vi "FTW-Reply-Worker.vi"(1 "Endpoint":refnum<class "FTW-Endpoint.lvclass">, 2 "Message Handler":refnum<user-event>) -> ()   [LabVIEW 2013, in "FTW-Reply.lvclass"]
uses:
  FTW-Reply.lvclass
  Package/Request/FTW-Package-IncomingRequest.lvclass
  Endpoint/FTW-Endpoint.lvclass
panel:
  out "Messages Handled":u32
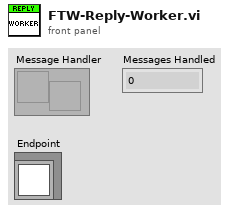
[diagram p1: front panel]
types:
  T1 = typedef "FTW-Message.ctl" = cluster{"Header":string, "Body":string, "Metadata":string}
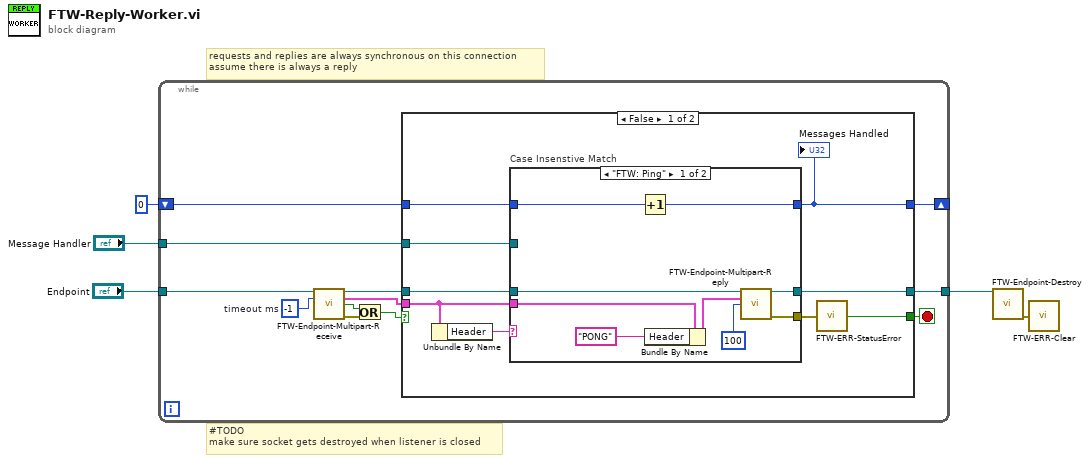
[diagram p0: block diagram]
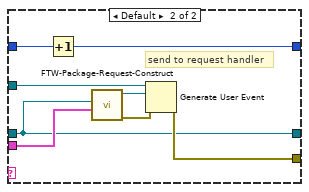
[diagram p2: hidden frame]
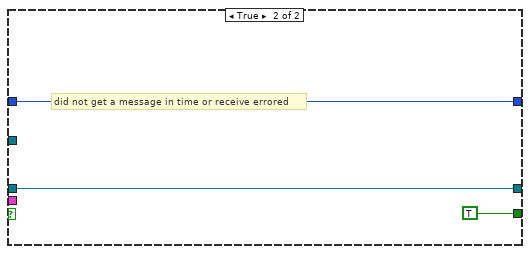
[diagram p3: hidden frame]
diagram:
  # "#TODO\nmake sure socket gets destroyed when listener is closed"
  # "requests and replies are always synchronous on this connection\nassume there is always a reply"
  n1 = while {
    tunnel: "Message Handler" -> [w17]
    shift-right: [w10] -> _
    shift-left: u32 0 -> [w11]
    tunnel: "Endpoint" -> [w16]
    tunnel: [w6] -> w3
    stop <- w12 stop-if-true
    w15 = -1  # timeout ms
    n2 = call-dynamic "FTW-Endpoint-Multipart-Receive.vi"("FTW Endpoint"=w16, "Timeout"=w15) -> ("FTW Endpoint out"=w9:refnum<class "FTW-Endpoint.lvclass">, "Message Received"=w13:T1, "Timed out?"=w7:bool, "error out"=w14:errorcluster)  [unwired: 10 in]
    n3 = Or(x=w7, y=w14) -> (x .or. y?=w8:bool)
    n4 = case shown="False" w8 {
      tunnel: w17 -> [w26 _]
      tunnel: w13 -> [w19 _]
      tunnel: [w22 TRUE] -> w12
      tunnel: w9 -> [w23 w44]
      tunnel: w11 -> [w25 w46]
      tunnel: [w20 w46] -> w10
      tunnel: [w21 w44] -> w6
      frame False {
        n5 = Unbundle By Name(w19) -> ("Header"=w18:string)
        n6 = case "Case Insenstive Match" shown="\"FTW: Ping\"" w18 {
          tunnel: w26 -> [_ w43]
          tunnel: w25 -> [w35 w42]
          tunnel: [w30 w41] -> w20
          tunnel: [w34 w38] -> w24
          tunnel: w23 -> [w33 w36]
          tunnel: w19 -> [w29 w37]
          tunnel: [w32 w36] -> w21
          frame "FTW: Ping" {
            n7 = Increment(x=w35) -> (x+1=w30:u32)
            n8 = Bundle By Name(cluster=w29, "Header"="PONG" ("Part")) -> (w28:T1)
            n9 = call-dynamic "FTW-Endpoint-Multipart-Reply.vi"("FTW Endpoint"=w33, "Message"=w28, "Timeout"=100) -> ("FTW Endpoint out"=w32:refnum<class "FTW-Endpoint.lvclass">, "error out"=w34:errorcluster)  [unwired: 10 in, 1 out]
          }
          frame Default {
            # "send to request handler"
            n10 = Increment(x=w42) -> (x+1=w41:u32)
            n11 = call "FTW-Package-Request-Construct.vi"("Message"=w37, "Frontend Endpoint"=w36) -> ("error out"=w40:errorcluster, "FTW Incoming Request"=w39:refnum<class "FTW-Package-IncomingRequest.lvclass">)  [unwired: 8 in]
            n12 = Generate User Event(user event=w43, event data cluster=w39, error in=w40) -> (error out=w38:errorcluster)  [unwired: 1 in, 1 out]
          }
        }
        "Messages Handled" <- w20
        n13 = call "FTW-ERR-StatusError.vi"("error to check"=w24) -> ("Error?"=w22:bool)
      }
      frame True {
        # "did not get a message in time or receive errored"
      }
    }
  }
  n14 = call-dynamic "FTW-Endpoint-Destroy.vi"("FTW Endpoint"=w3) -> ("error out"=w1:errorcluster)  [unwired: 14 in]
  n15 = call "FTW-ERR-Clear.vi"("error to snuff"=w1) -> ()  [unwired: 1 out]
